vi "calculate track length.vi"(9 "Measures":i32, 10 "BPM":i32, 11 "Enum":enum16{"4/4", "3/4"}(ring)=enum."3/4") -> (0 "total number of beats":i32, 1 "bps":dbl, 3 "Track Length (s)":dbl format="%.2f")   [LabVIEW 2014]
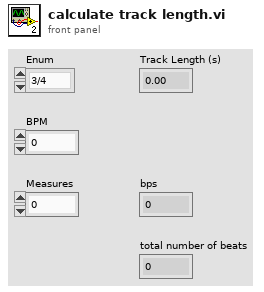
[diagram p1: front panel]
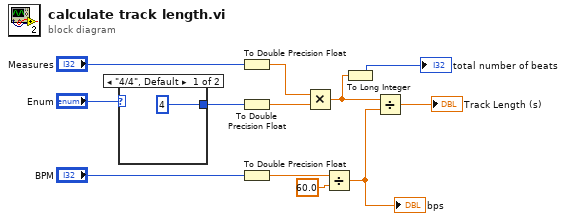
[diagram p0: block diagram]
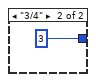
[diagram p2: hidden frame]
diagram:
  n1 = case shown="\"4/4\", Default" "Enum" {
    tunnel: [4 ("1 minute") 3 ("1 minute")] -> w11
    frame "4/4", Default {
    }
    frame "3/4" {
    }
  }
  n2 = To Double Precision Float(number="Measures") -> (double precision float=w6:dbl)
  n3 = To Double Precision Float(number=w11) -> (double precision float=w5:dbl)
  n4 = To Double Precision Float(number="BPM") -> (double precision float=w8:dbl)
  n5 = Multiply(x=w6, y=w5) -> (x*y=w2:dbl)
  n6 = Divide(x=w8, y=60.0) -> (x/y=w4:dbl)
  "bps" <- w4
  n7 = To Long Integer(number=w2) -> (32bit integer=→"total number of beats":i32)
  n8 = Divide(x=w2, y=w4) -> (x/y=→"Track Length (s)":dbl)
